vi "Search Real Numbers with Approximation.vi"(10 "tolerance for real numbers":dbl=1e-10, 11 "Numbers":cdb[](array[numeric])) -> (2 "Real Numbers":dbl[](array[numeric]), 3 "Complex Numbers":cdb[](array[numeric]))   [LabVIEW 2020, in "NI_AALPro.lvlib"]
uses:
  NI_AALPro.lvlib
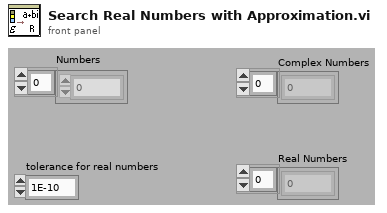
[diagram p1: front panel]
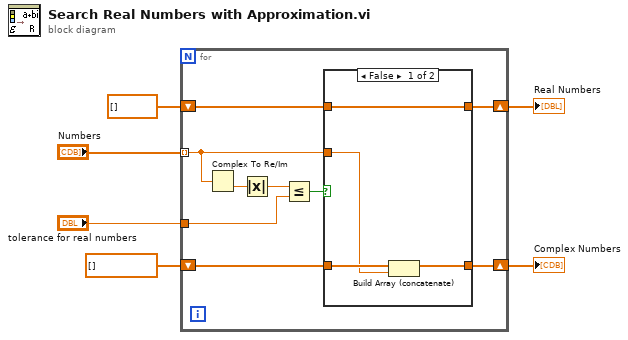
[diagram p0: block diagram]
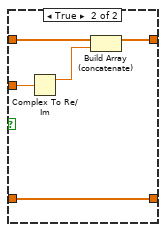
[diagram p2: hidden frame]
diagram:
  n1 = for {
    tunnel: "Numbers" -> [w12] mode=indexing
    shift-right: [w8] -> w2
    shift-left: dbl[] [] ("BDL") -> [w14]
    shift-right: [w7] -> w1
    shift-left: cdb[] [] ("CDB") -> [w13]
    tunnel: "tolerance for real numbers" -> [w10]
    n2 = Complex To Re/Im(x + iy=w12) -> (y=w15:dbl)  [unwired: 1 out]
    n3 = Absolute Value(x=w15) -> (abs(x)=w11:dbl)
    n4 = Less Or Equal?(x=w11, y=w10) -> (x <= y?=w9:bool)
    n5 = case shown="False" w9 {
      tunnel: w14 -> [w19 w23]
      tunnel: w13 -> [w18 w20]
      tunnel: w12 -> [w17 w24]
      tunnel: [w19 w22] -> w8
      tunnel: [w16 w20] -> w7
      frame False {
        n6 = Build Array (concatenate)(w18, w17) -> (w16:cdb[])
      }
      frame True {
        n7 = Complex To Re/Im(x + iy=w24) -> (x=w21:dbl)  [unwired: 1 out]
        n8 = Build Array (concatenate)(w23, w21) -> (w22:dbl[])
      }
    }
  }
  "Real Numbers" <- w2
  "Complex Numbers" <- w1
